vi "Bank Tester.vi"(8 "error in (no error)":errorcluster) -> (0 "error out":errorcluster)   [LabVIEW 2010]
uses:
  Account Info.ctl
  Stop.vi
panel:
  in  "Command":T1
  in  "Deposit Amount":dbl
  in  "Withdrawal Amount":dbl
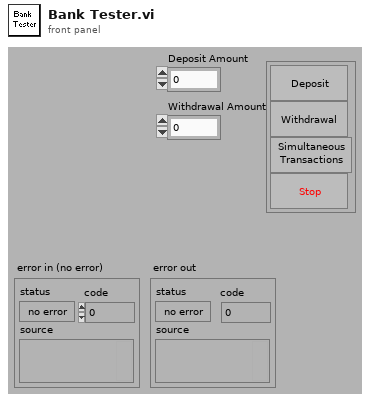
[diagram p1: front panel]
types:
  T1 = cluster{"Deposit":bool, "Withdrawl":bool, "Simultaneous":bool, "Simultaneous 2":bool}
  T2 = typedef "Account Info.ctl" = cluster{"Bank Rendezvous":T3, "Withdrawal Queue":refnum<queue>, "Deposit Queue":refnum<queue>}
  T3 = typedef "Rendezvous RefNum" = refnum<k1>
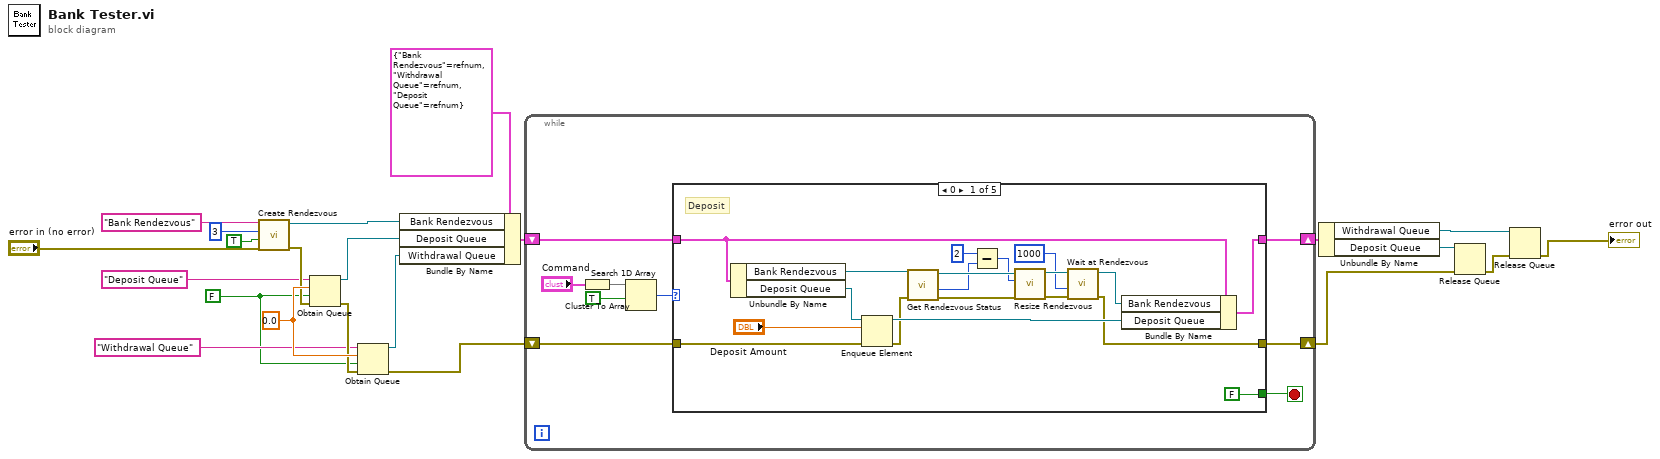
[diagram p0: block diagram]
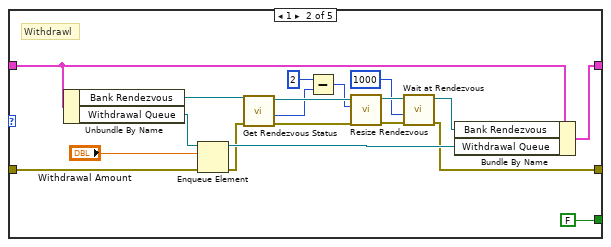
[diagram p2: hidden frame]
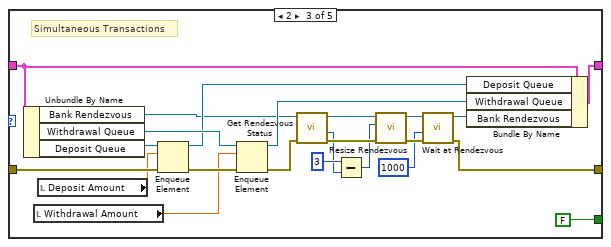
[diagram p3: hidden frame]
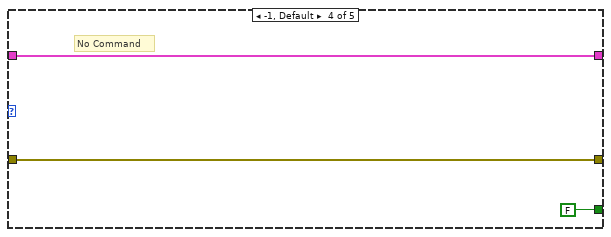
[diagram p4: hidden frame]
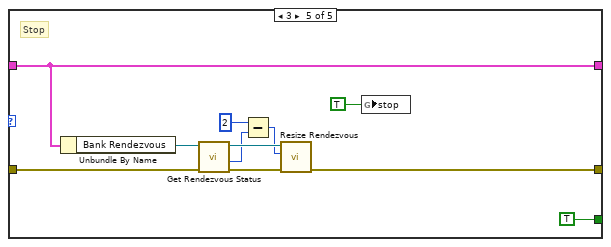
[diagram p5: hidden frame]
diagram:
  w1 = FALSE ("return existing (F)")
  w21 = 0.0
  n1 = call <vilib>:"Create Rendezvous.vi"("error in (no error)"="error in (no error)", "return existing (F)"=TRUE, "size (2)"=3, "name (unnamed)"="Bank Rendezvous") -> ("error out"=w20:errorcluster, "rendezvous"=w22:T3)  [unwired: 1 in, 1 out]
  n2 = Obtain Queue(name (unnamed)="Deposit Queue", element data type=w21, create if not found? (T)=w1, error in (no error)=w20) -> (queue out=w18:refnum<queue>, error out=w19:errorcluster)  [unwired: 1 in, 1 out]
  n3 = Obtain Queue(name (unnamed)="Withdrawal Queue", element data type=w21, create if not found? (T)=w1, error in (no error)=w19) -> (queue out=w17:refnum<queue>, error out=w9:errorcluster)  [unwired: 1 in, 1 out]
  n4 = Bundle By Name(cluster=T2 {"Bank Rendezvous"=refnum, "Withdrawal Queue"=refnum, "Deposit Queue"=refnum}, "Bank Rendezvous"=w22, "Deposit Queue"=w18, "Withdrawal Queue"=w17) -> (w11:T2)
  n5 = while {
    shift-right: [w25] -> w4
    shift-left: w9 -> [w24]
    shift-right: [w26] -> w8
    shift-left: w11 -> [w28]
    stop <- w23 stop-if-true
    n6 = Cluster To Array(cluster="Command") -> (array=w30:bool[])
    n7 = Search 1D Array(1D array=w30, element=TRUE) -> (index of element=w29:i32)  [unwired: 1 in]
    n8 = case shown="0" w29 {
      tunnel: w28 -> [w42 w62 w88 w95 w104]
      tunnel: w24 -> [w48 w68 w85 w94 w100]
      tunnel: [w43 w63 w89 w95 w104] -> w26
      tunnel: [w41 w61 w87 w94 w96] -> w25
      tunnel: [FALSE FALSE FALSE FALSE TRUE] -> w23
      frame 0 {
        # "Deposit"
        n9 = Unbundle By Name(w42) -> ("Bank Rendezvous"=w36:T3, "Deposit Queue"=w50:refnum<queue>)
        n10 = Enqueue Element(queue=w50, element="Deposit Amount", error in (no error)=w48) -> (queue out=w44:refnum<queue>, error out=w38:errorcluster)  [unwired: 1 in, 1 out]
        n11 = call <vilib>:"Get Rendezvous Status.vi"("error in (no error)"=w38, "rendezvous"=w36) -> ("error out"=w37:errorcluster, "size"=w33:i32, "rendezvous out"=w35:T3)  [unwired: 5 in, 2 out]
        n12 = Subtract(x=2 ("size change (0)"), y=w33) -> (x-y=w32:i32)
        n13 = call <vilib>:"Resize Rendezvous.vi"("error in (no error)"=w37, "size change (0)"=w32, "rendezvous"=w35) -> ("error out"=w47:errorcluster, "rendezvous out"=w46:T3)  [unwired: 2 in, 1 out]
        n14 = call <vilib>:"Wait at Rendezvous.vi"("error in (no error)"=w47, "ms timeout (-1)"=1000, "rendezvous"=w46) -> ("error out"=w41:errorcluster, "rendezvous out"=w45:T3)  [unwired: 2 in, 1 out]
        n15 = Bundle By Name(cluster=w42, "Bank Rendezvous"=w45, "Deposit Queue"=w44) -> (w43:T2)
      }
      frame 1 {
        # "Withdrawl"
        n16 = Unbundle By Name(w62) -> ("Bank Rendezvous"=w56:T3, "Withdrawal Queue"=w69:refnum<queue>)
        n17 = Enqueue Element(queue=w69, element="Withdrawal Amount", error in (no error)=w68) -> (queue out=w64:refnum<queue>, error out=w58:errorcluster)  [unwired: 1 in, 1 out]
        n18 = call <vilib>:"Get Rendezvous Status.vi"("error in (no error)"=w58, "rendezvous"=w56) -> ("error out"=w57:errorcluster, "size"=w53:i32, "rendezvous out"=w55:T3)  [unwired: 5 in, 2 out]
        n19 = Subtract(x=2 ("size change (0)"), y=w53) -> (x-y=w52:i32)
        n20 = call <vilib>:"Resize Rendezvous.vi"("error in (no error)"=w57, "size change (0)"=w52, "rendezvous"=w55) -> ("error out"=w67:errorcluster, "rendezvous out"=w66:T3)  [unwired: 2 in, 1 out]
        n21 = call <vilib>:"Wait at Rendezvous.vi"("error in (no error)"=w67, "ms timeout (-1)"=1000, "rendezvous"=w66) -> ("error out"=w61:errorcluster, "rendezvous out"=w65:T3)  [unwired: 2 in, 1 out]
        n22 = Bundle By Name(cluster=w62, "Bank Rendezvous"=w65, "Withdrawal Queue"=w64) -> (w63:T2)
      }
      frame 2 {
        # "Simultaneous Transactions"
        n23 = Unbundle By Name(w88) -> ("Bank Rendezvous"=w76:T3, "Withdrawal Queue"=w92:refnum<queue>, "Deposit Queue"=w86:refnum<queue>)
        n24 = local read "Withdrawal Amount"() -> (w79:dbl)
        n25 = local read "Deposit Amount"() -> (w80:dbl)
        n26 = Enqueue Element(queue=w86, element=w80, error in (no error)=w85) -> (queue out=w83:refnum<queue>, error out=w84:errorcluster)  [unwired: 1 in, 1 out]
        n27 = Enqueue Element(queue=w92, element=w79, error in (no error)=w84) -> (queue out=w81:refnum<queue>, error out=w75:errorcluster)  [unwired: 1 in, 1 out]
        n28 = call <vilib>:"Get Rendezvous Status.vi"("error in (no error)"=w75, "rendezvous"=w76) -> ("error out"=w74:errorcluster, "size"=w71:i32, "rendezvous out"=w73:T3)  [unwired: 5 in, 2 out]
        n29 = Subtract(x=3 ("size change (0)"), y=w71) -> (x-y=w70:i32)
        n30 = call <vilib>:"Resize Rendezvous.vi"("error in (no error)"=w74, "size change (0)"=w70, "rendezvous"=w73) -> ("error out"=w91:errorcluster, "rendezvous out"=w90:T3)  [unwired: 2 in, 1 out]
        n31 = call <vilib>:"Wait at Rendezvous.vi"("error in (no error)"=w91, "ms timeout (-1)"=1000, "rendezvous"=w90) -> ("error out"=w87:errorcluster, "rendezvous out"=w82:T3)  [unwired: 2 in, 1 out]
        n32 = Bundle By Name(cluster=w88, "Deposit Queue"=w83, "Withdrawal Queue"=w81, "Bank Rendezvous"=w82) -> (w89:T2)
      }
      frame -1, Default {
        # "No Command"
      }
      frame 3 {
        # "Stop"
        n33 = Unbundle By Name(w104) -> ("Bank Rendezvous"=w101:T3)
        n34 = call <vilib>:"Get Rendezvous Status.vi"("error in (no error)"=w100, "rendezvous"=w101) -> ("error out"=w103:errorcluster, "size"=w99:i32, "rendezvous out"=w102:T3)  [unwired: 5 in, 2 out]
        n35 = Subtract(x=2, y=w99) -> (x-y=w97:i32)
        n36 = call <vilib>:"Resize Rendezvous.vi"("error in (no error)"=w103, "size change (0)"=w97, "rendezvous"=w102) -> ("error out"=w96:errorcluster)  [unwired: 2 in, 2 out]
        n37 = global write "Stop.vi" "stop"(TRUE ("stop")) -> ()
      }
    }
  }
  n38 = Unbundle By Name(w8) -> ("Withdrawal Queue"=w6:refnum<queue>, "Deposit Queue"=w7:refnum<queue>)
  n39 = Release Queue(queue=w7, error in (no error)=w4) -> (error out=w5:errorcluster)  [unwired: 1 in, 2 out]
  n40 = Release Queue(queue=w6, error in (no error)=w5) -> (error out=→"error out":errorcluster)  [unwired: 1 in, 2 out]
